vi "DAQ.vi"() -> ()   [LabVIEW 2014]
uses:
  <vilib>/LabVIEW Open Source Project/MQTT Control Packets/Control Packets/CONNECT/ConnectFlags -- cluster.ctl
  <vilib>/LabVIEW Open Source Project/MQTT Client/Client class/Client.lvclass/Client.ctl
  <vilib>/LabVIEW Open Source Project/MQTT Connection/MQTT_Base/Base Class/MQTT_Base.lvclass/MQTT_Base.ctl
  <vilib>/Utility/error.llb/Error Cluster From Error Code.vi
  <vilib>/LabVIEW Open Source Project/MQTT Control Packets/Control Packets/PUBLISH/PUBLISH.lvclass
  <vilib>/LabVIEW Open Source Project/MQTT Client/Client class/Client.lvclass
  <vilib>/ErrorRing/Error Ring.xnode
  <vilib>/LabVIEW Open Source Project/MQTT Connection/MQTT_Base/Base Class/MQTT_Base.lvclass
  <vilib>/LabVIEW Open Source Project/MQTT TCP Connection/MQTT_TCP/Connection/TCPConnection.lvclass
  <vilib>/LabVIEW Open Source Project/MQTT Control Packets/Control Packets/CONNECT/CONNECT.lvclass
panel:
  out "Array":string[](array[string])
  out "Data from subscribe":string
  out "Array 3":bool[](array[boolean])
  out "Time":u32
  in  "MQTT":enum32{"MQTT configs", "Equipment"}(tab)
  in  "Connect Flags":T1[](array[typedef])=[{"Reserved"=FALSE, "Clean Session"=FALSE, "Will Flag"=FALSE, "Will QoS 1"=FALSE, "Will QoS 2"=FALSE, "Will Retain"=FALSE, "Password Flag"=FALSE, "User Name Flag"=TRUE}, {"Reserved"=FALSE, "Clean Session"=FALSE, "Will Flag"=FALSE, "Will QoS 1"=FALSE, "Will QoS 2"=FALSE, "Will Retain"=FALSE, "Password Flag"=FALSE, "User Name Flag"=TRUE}, {"Reserved"=FALSE, "Clean Session"=FALSE, "Will Flag"=FALSE, "Will QoS 1"=FALSE, "Will QoS 2"=FALSE, "Will Retain"=FALSE, "Password Flag"=FALSE, "User Name Flag"=TRUE}, {"Reserved"=FALSE, "Clean Session"=FALSE, "Will Flag"=FALSE, "Will QoS 1"=FALSE, "Will QoS 2"=FALSE, "Will Retain"=FALSE, "Password Flag"=FALSE, "User Name Flag"=TRUE}, {"Reserved"=FALSE, "Clean Session"=FALSE, "Will Flag"=FALSE, "Will QoS 1"=FALSE, "Will QoS 2"=FALSE, "Will Retain"=FALSE, "Password Flag"=FALSE, "User Name Flag"=TRUE}, {"Reserved"=FALSE, "Clean Session"=FALSE, "Will Flag"=FALSE, "Will QoS 1"=FALSE, "Will QoS 2"=FALSE, "Will Retain"=FALSE, "Password Flag"=FALSE, "User Name Flag"=TRUE}]
  in  "User Devices":T2(array[cluster])=[{"Will Topic"="v1/devices/me/telemetry", "Will Message"="", "Username"="Valve-01", "Password"=""}, {"Will Topic"="v1/devices/me/telemetry", "Will Message"="", "Username"="Valve-02", "Password"=""}, {"Will Topic"="v1/devices/me/telemetry", "Will Message"="", "Username"="PP-01", "Password"=""}, {"Will Topic"="v1/devices/me/telemetry", "Will Message"="", "Username"="Level-01", "Password"=""}, {"Will Topic"="v1/devices/me/telemetry", "Will Message"="", "Username"="QT-01", "Password"=""}, {"Will Topic"="v1/devices/me/telemetry", "Will Message"="", "Username"="QT-02", "Password"=""}]
  in  "address (localhost)":string="things.ktk.gubkin.ru"
  in  "remote port (80)":u16=1883
  in  "PVs":string[](array[string])=["AI_rOpen_vlv1", "AI_rOpen_vlv2", "RA_rCntrl_engine_S", "AI_rlvl", "PV_AIFLOW1", "PV_AIFLOW2"]
  in  "OPs":string[](array[string])=["RA_rCntrl_vlv1_S", "RA_rCntrl_vlv2_S", "RA_rCntrl_engine_S"]
  out "error out":errorcluster
  in  "Frequency":dbl=10.0
  out "Display":string
  in  "Stop":bool
  in  "Exit":bool
  in  "Start":bool
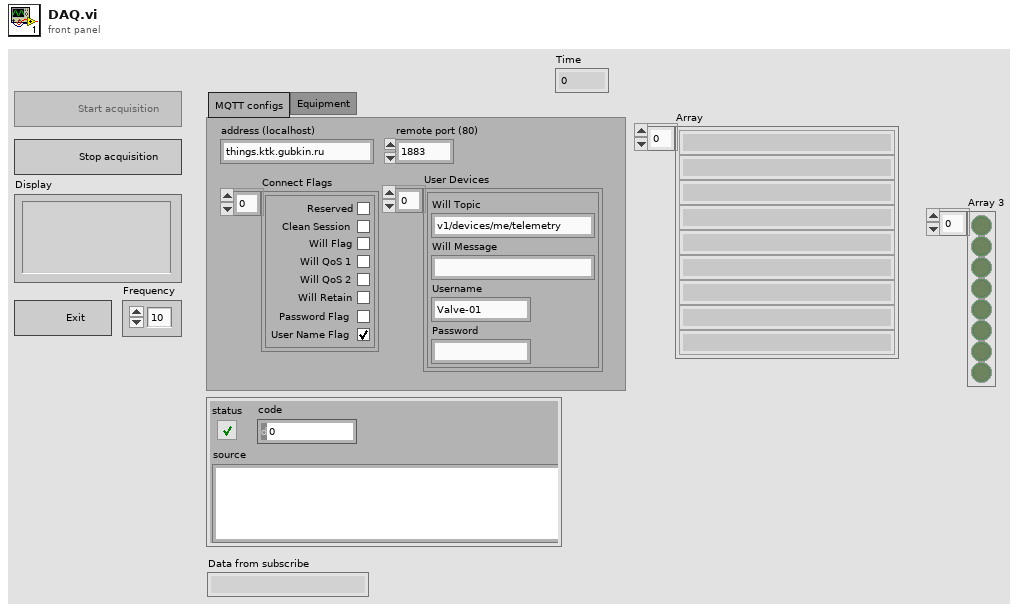
[diagram p1: front panel]
types:
  T1 = typedef "MQTT_Control_Packets.lvlib/CONNECT.lvclass/ConnectFlags -- cluster.ctl" = cluster{"Reserved":bool, "Clean Session":bool, "Will Flag":bool, "Will QoS 1":bool, "Will QoS 2":bool, "Will Retain":bool, "Password Flag":bool, "User Name Flag":bool}
  T2 = cluster{"Will Topic":string, "Will Message":string, "Username":string, "Password":string}[]
  T3 = cluster{"Start":refnum<vi>, "Stop":refnum<vi>, "Display":refnum<vi>, "Exit":refnum<vi>}
  T4 = cluster{"UI":refnum<queue>, "Acquisition":refnum<queue>}
  T5 = enum8{"Enabled", "Disabled", "Disabled and Grayed Out"}
  T6 = enum16{"Read", "Write", "ReadWrite", "BufferedRead", "BufferedReadWrite"}
  T7 = typedef "MQTT Client.lvlib/Client.lvclass/Public Events -- cluster.ctl" = cluster{"Connection Status":refnum<user-event>, "Connected":refnum<user-event>, "Application Message":refnum<user-event>}
  T8 = typedef "MQTT Base.lvlib/MQTT_Base.lvclass/Public Events -- cluster.ctl" = cluster{"Stop Event":refnum<user-event>, "Error Event":refnum<user-event>, "Inbound Message":refnum<user-event>}
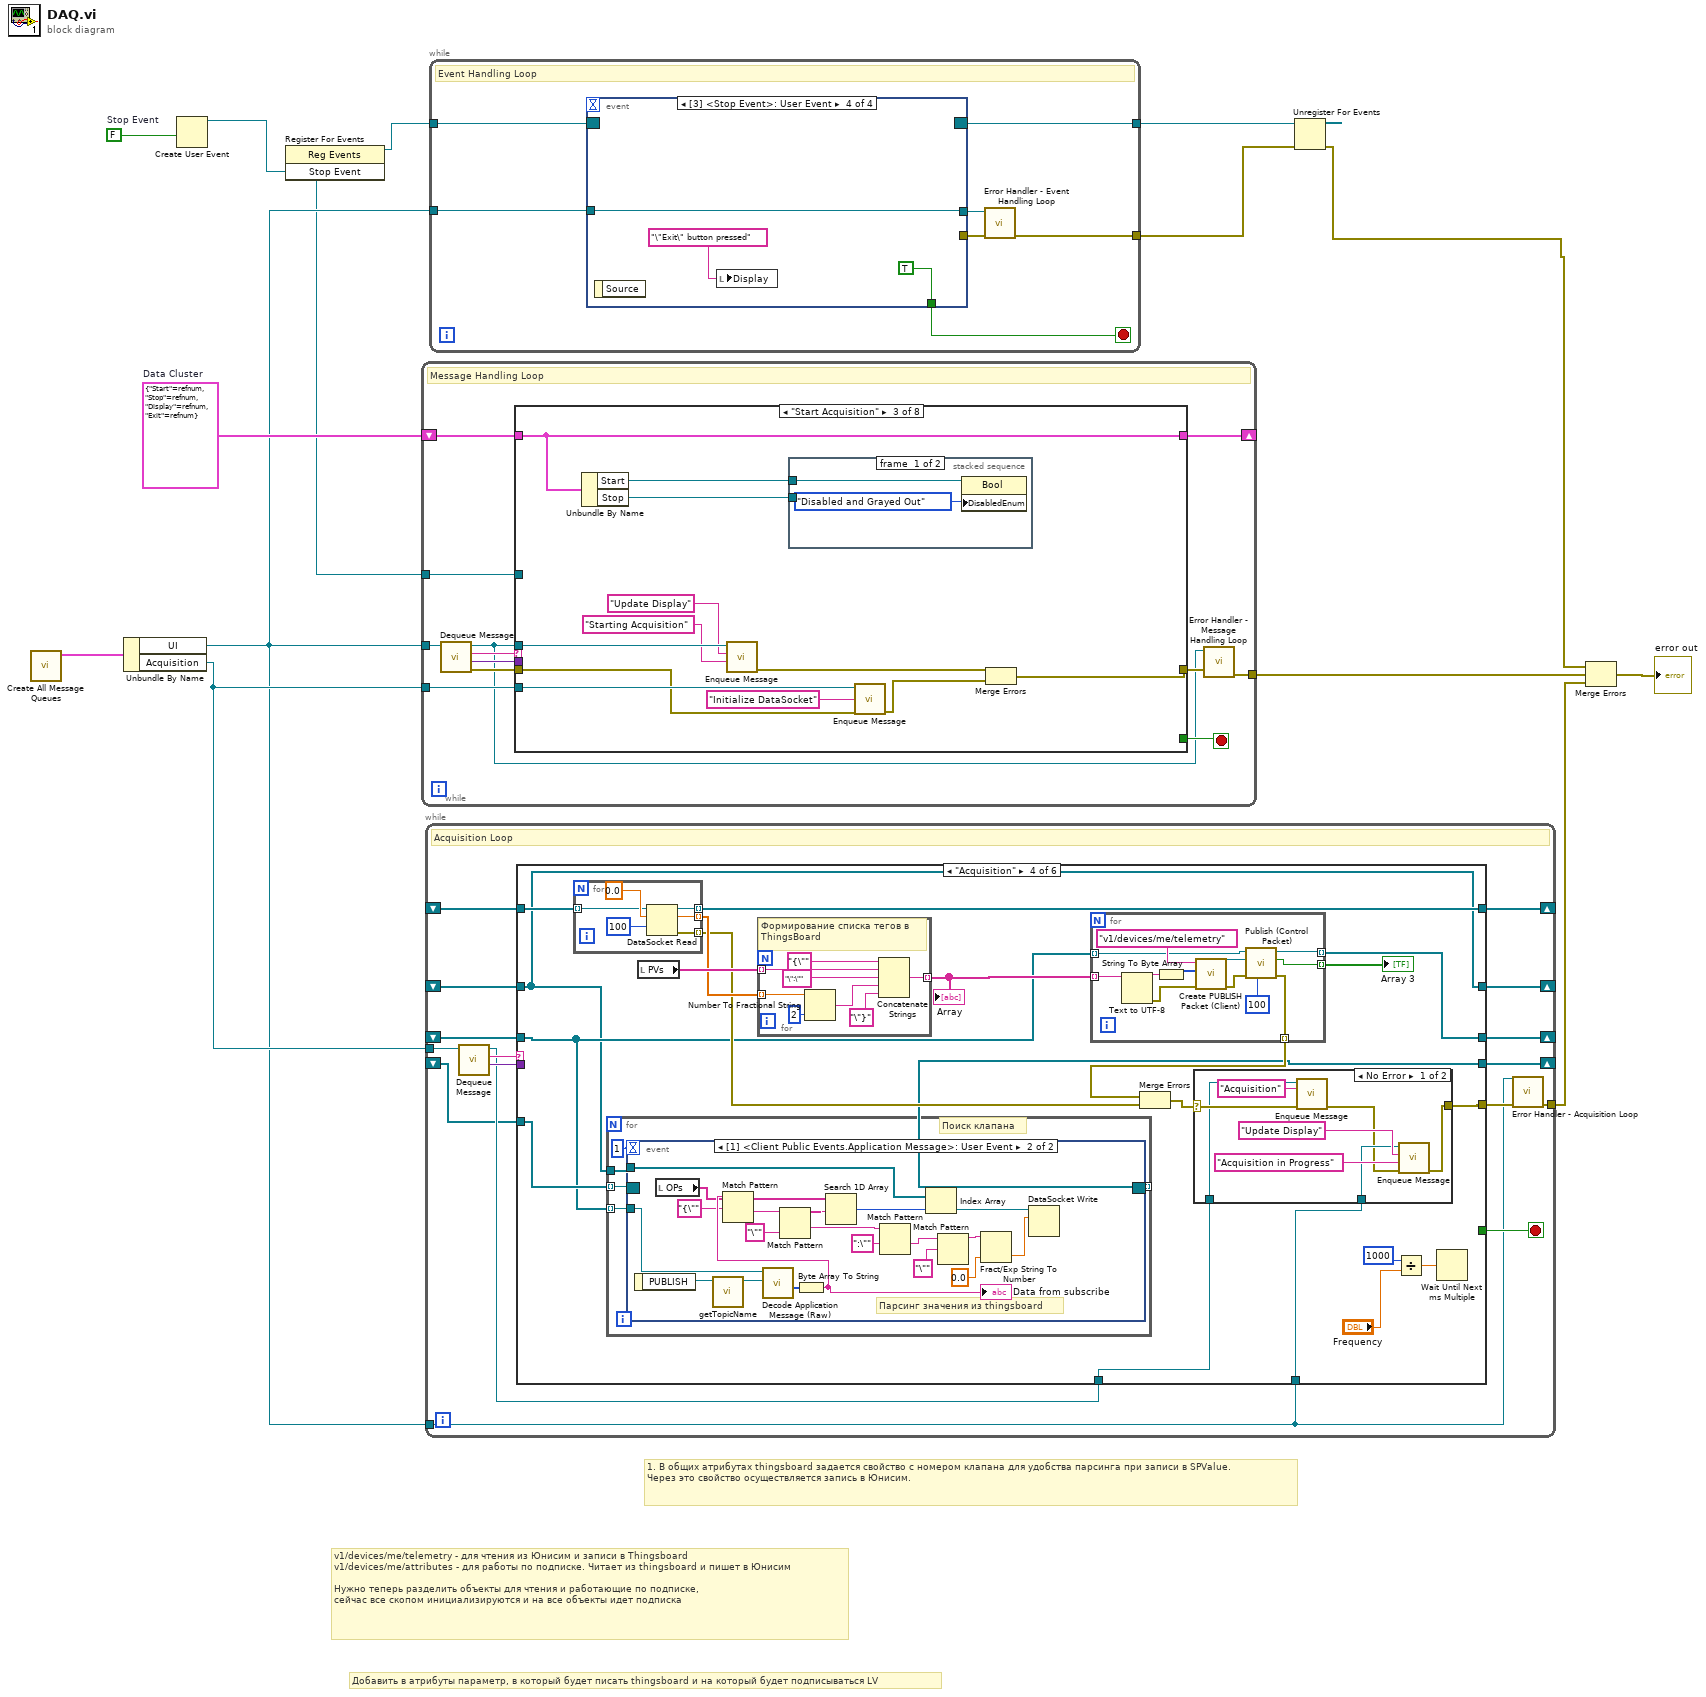
[diagram p0: block diagram]
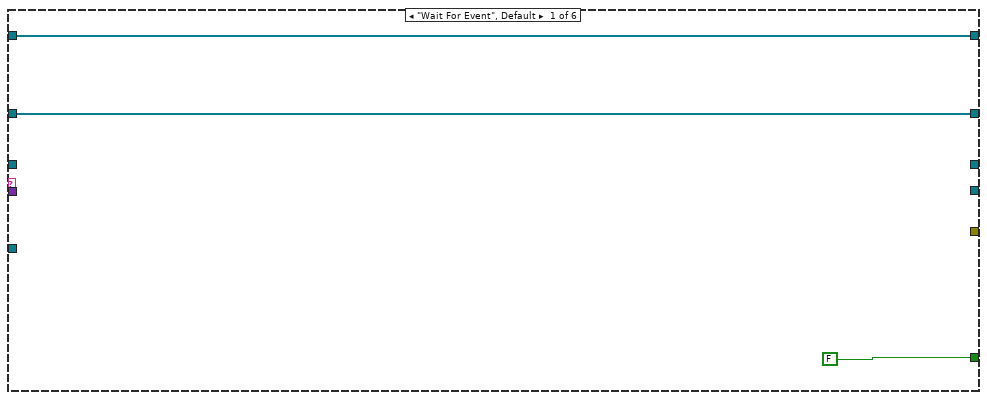
[diagram p2: hidden frame]
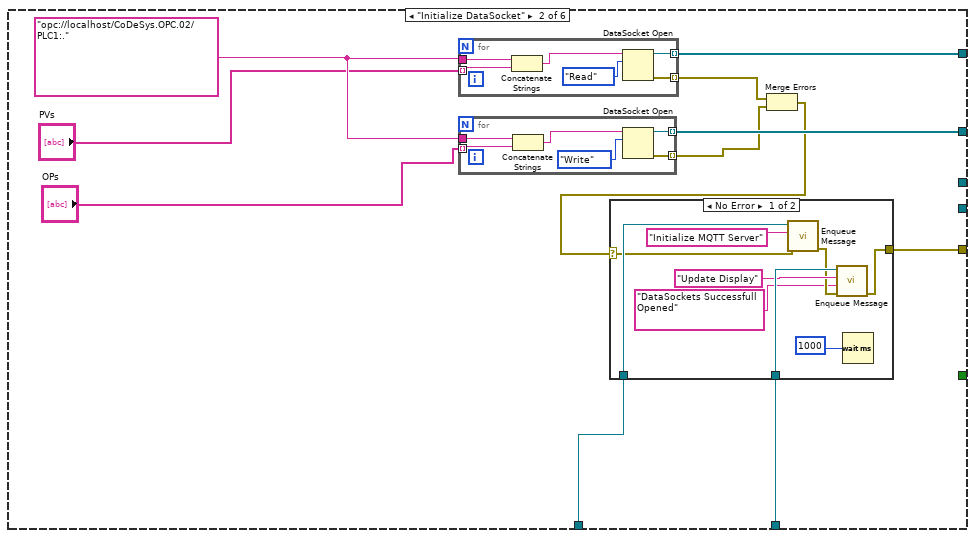
[diagram p3: hidden frame]
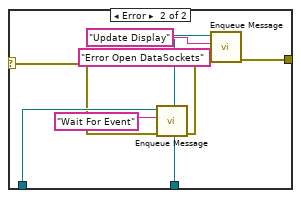
[diagram p4: hidden frame]
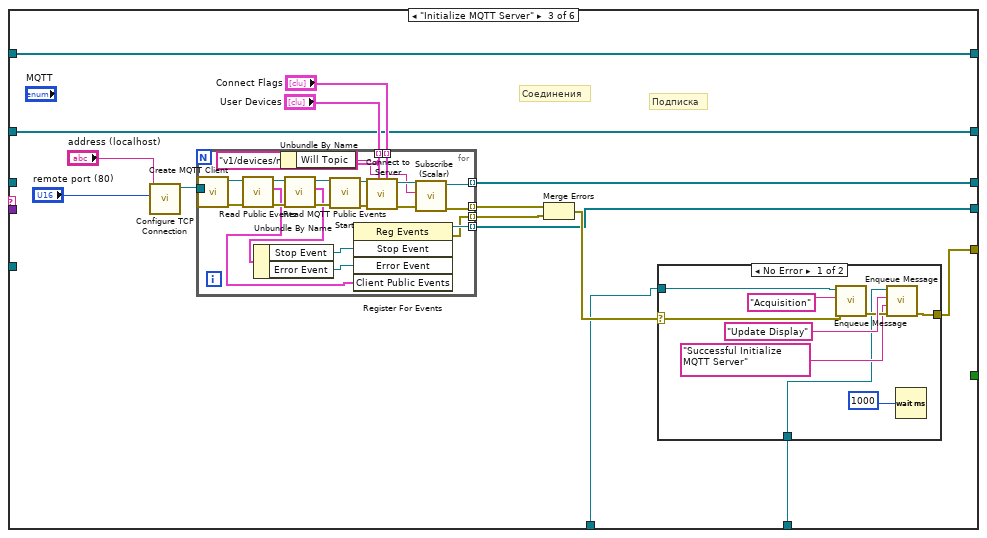
[diagram p5: hidden frame]
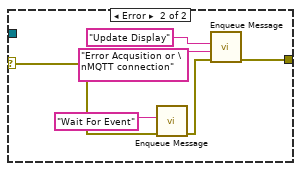
[diagram p6: hidden frame]
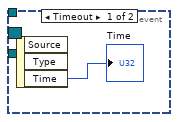
[diagram p7: hidden frame]
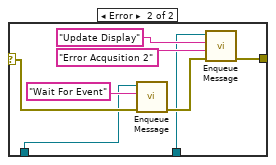
[diagram p8: hidden frame]
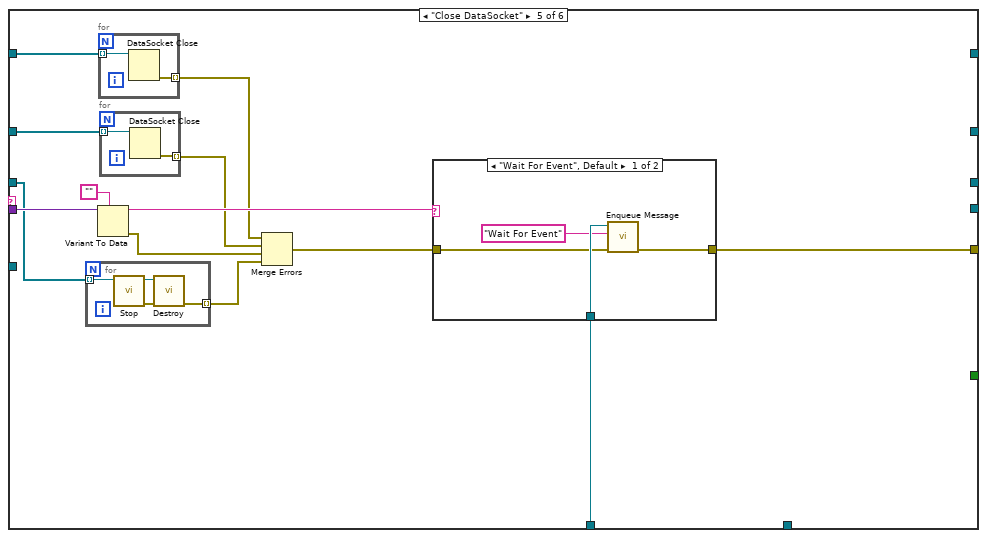
[diagram p9: hidden frame]
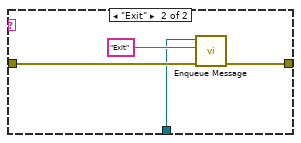
[diagram p10: hidden frame]
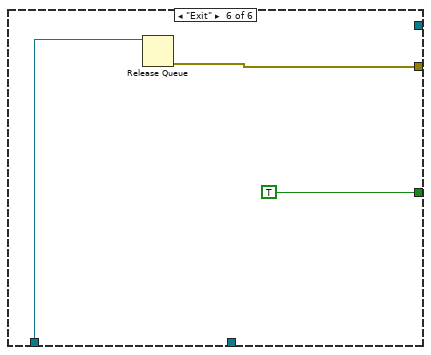
[diagram p11: hidden frame]
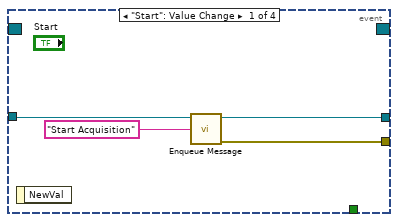
[diagram p12: hidden frame]
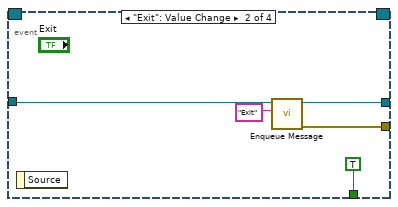
[diagram p13: hidden frame]
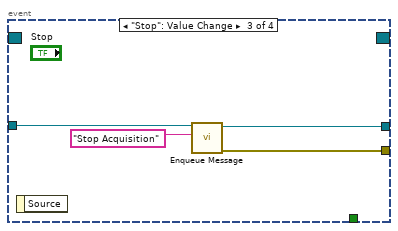
[diagram p14: hidden frame]
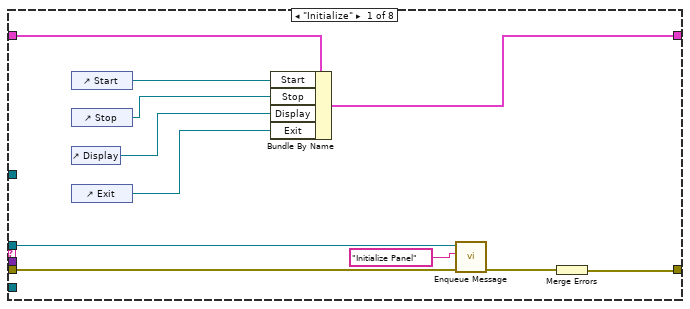
[diagram p15: hidden frame]
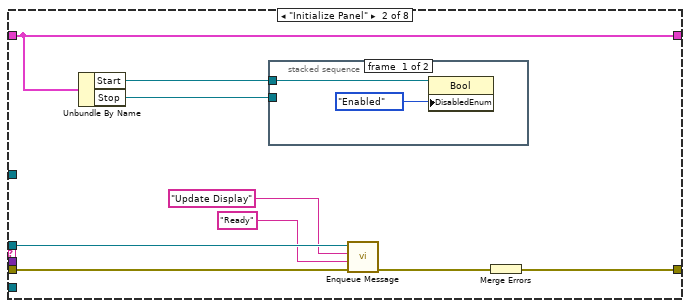
[diagram p16: hidden frame]
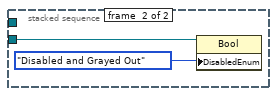
[diagram p17: hidden frame]
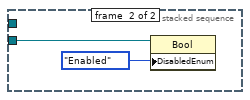
[diagram p18: hidden frame]
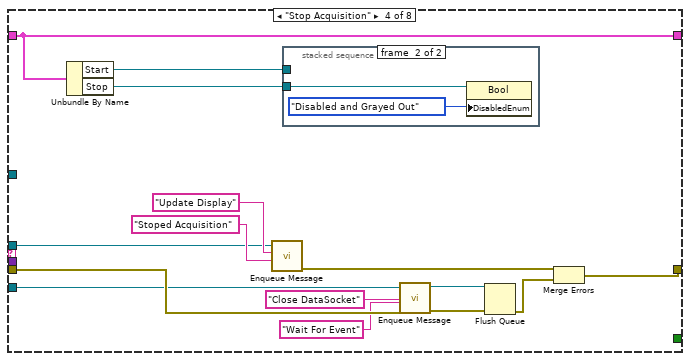
[diagram p19: hidden frame]
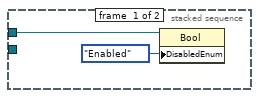
[diagram p20: hidden frame]
diagram:
  w7 = FALSE  # Stop Event
  w12 = T3 {"Start"=refnum, "Stop"=refnum, "Display"=refnum, "Exit"=refnum}  # Data Cluster
  # "1. В общих атрибутах thingsboard задается свойство с номером клапана для удобства парсинга при записи в SPValue.\nЧерез это свойство осуществляется запись в Юнисим."
  # "Добавить в атрибуты параметр, в который будет писать thingsboard и на который будет подписываться LV"
  # "v1/devices/me/telemetry - для чтения из Юнисим и записи в Thingsboard\nv1/devices/me/attributes - для работы по подписке. Читает из thingsboard и пишет в Юнисим\n\nНужно теперь разделить объекты для чтения и работающие по подписке,\nсейчас все скопом инициализируются и на все объекты идет подписка"
  n1 = call "Create All Message Queues.vi"() -> ("Message Queues out"=w13:T4)  [unwired: 10 in, 1 out]
  n2 = Unbundle By Name(w13) -> ("UI"=w10:refnum<queue>, "Acquisition"=w11:refnum<queue>)
  n3 = Create User Event(user event datatype=w7) -> (user event=w6:refnum<user-event>)  [unwired: 1 in, 1 out]
  n4 = register-events(w6) -> (reference out=w5:refnum<event-registration>)  [unwired: 2 in, 1 out]
  n5 = while {
    tunnel: w10 -> [w24]
    shift-right: [w22] -> _
    shift-left: w12 -> [w18]
    tunnel: w11 -> [w21]
    tunnel: [w16] -> w9
    tunnel: w6 -> [w14]
    stop <- w19 stop-if-true
    # "Message Handling Loop"
    n6 = call "Dequeue Message.vi"("Queue in"=w24) -> ("error out"=w23:errorcluster, "Message Data"=w20:variant, "Message"=w25:string, "Queue out"=w15:refnum<queue>)  [unwired: 7 in]
    n7 = case shown="\"Start Acquisition\"" w25 {
      selector: w25 -> [_ _ _ _ _ _ _ w121]
      tunnel: w18 -> [w36 w44 w61 w80 w88 w93 w115 w122]
      tunnel: w15 -> [w31 w43 w58 w73 _ w98 w112 _]
      tunnel: w23 -> [w30 w42 w51 w72 w89 w100 w111 _]
      tunnel: [w28 w44 w61 w80 w88 w93 w115 w122] -> w22
      tunnel: w21 -> [_ _ w55 w71 _ _ w110 _]
      tunnel: w20 -> [_ _ _ _ w90 w101 _ _]
      tunnel: [_ _ _ _ _ _ TRUE _] -> w19
      tunnel: [w26 w37 w50 w66 w85 w92 w104 w120] -> w17
      tunnel: w14 -> [_ _ _ _ _ _ w103 _]
      frame "Initialize" {
        n8 = control-ref of="Start"() -> (w35:refnum<vi>)
        n9 = control-ref of="Stop"() -> (w34:refnum<vi>)
        n10 = control-ref of="Display"() -> (w33:refnum<vi>)
        n11 = control-ref of="Exit"() -> (w32:refnum<vi>)
        n12 = Bundle By Name(cluster=w36, "Start"=w35, "Stop"=w34, "Display"=w33, "Exit"=w32) -> (w28:T3)
        n13 = call "Enqueue Message.vi"("error in (no error)"=w30, "Message"="Initialize Panel", "Queue in"=w31) -> ("error out"=w27:errorcluster)  [unwired: 7 in, 1 out]
        n14 = Merge Errors(w27) -> (w26:errorcluster)
      }
      frame "Initialize Panel" {
        n15 = Unbundle By Name(w44) -> ("Start"=w38:refnum<vi>, "Stop"=w45:refnum<vi>)
        n16 = stacked-sequence {
          tunnel: w38 -> [w47 _]
          tunnel: w45 -> [_ w48]
          frame #0 {
            n17 = property class="Bool"(reference=w47, "DisabledEnum"=T5."Enabled" ("Disabled")) -> ()  [unwired: 1 in, 2 out]
          }
          frame #1 {
            n18 = property class="Bool"(reference=w48, "DisabledEnum"=T5."Disabled and Grayed Out" ("Disabled")) -> ()  [unwired: 1 in, 2 out]
          }
        }
        n19 = call "Enqueue Message.vi"("error in (no error)"=w42, "Message Data"="Ready" ("Message"), "Message"="Update Display", "Queue in"=w43) -> ("error out"=w39:errorcluster)  [unwired: 6 in, 1 out]
        n20 = Merge Errors(w39) -> (w37:errorcluster)
      }
      frame "Start Acquisition" {
        n21 = Unbundle By Name(w61) -> ("Start"=w60:refnum<vi>, "Stop"=w59:refnum<vi>)
        n22 = call "Enqueue Message.vi"("Message Data"="Starting Acquisition" ("Message"), "Message"="Update Display", "Queue in"=w58) -> ("error out"=w53:errorcluster)  [unwired: 7 in, 1 out]
        n23 = stacked-sequence {
          tunnel: w60 -> [w62 _]
          tunnel: w59 -> [_ w64]
          frame #0 {
            n24 = property class="Bool"(reference=w62, "DisabledEnum"=T5."Disabled and Grayed Out" ("Disabled")) -> ()  [unwired: 1 in, 2 out]
          }
          frame #1 {
            n25 = property class="Bool"(reference=w64, "DisabledEnum"=T5."Enabled" ("Disabled")) -> ()  [unwired: 1 in, 2 out]
          }
        }
        n26 = call "Enqueue Message.vi"("error in (no error)"=w51, "Message"="Initialize DataSocket", "Queue in"=w55) -> ("error out"=w52:errorcluster)  [unwired: 7 in, 1 out]
        n27 = Merge Errors(w53, w52) -> (w50:errorcluster)
      }
      frame "Stop Acquisition" {
        n28 = Unbundle By Name(w80) -> ("Start"=w79:refnum<vi>, "Stop"=w78:refnum<vi>)
        n29 = call "Enqueue Message.vi"("Message Data"="Stoped Acquisition" ("Message"), "Message"="Update Display", "Queue in"=w73) -> ("error out"=w77:errorcluster)  [unwired: 7 in, 1 out]
        n30 = stacked-sequence {
          tunnel: w79 -> [w81 _]
          tunnel: w78 -> [_ w83]
          frame #0 {
            n31 = property class="Bool"(reference=w81, "DisabledEnum"=T5."Enabled" ("Disabled")) -> ()  [unwired: 1 in, 2 out]
          }
          frame #1 {
            n32 = property class="Bool"(reference=w83, "DisabledEnum"=T5."Disabled and Grayed Out" ("Disabled")) -> ()  [unwired: 1 in, 2 out]
          }
        }
        n33 = call "Enqueue Message.vi"("error in (no error)"=w72, "Message Data"="Wait For Event" ("Message"), "Message"="Close DataSocket", "Queue in"=w71) -> ("error out"=w68:errorcluster, "Queue out"=w69:refnum<queue>)  [unwired: 6 in]
        n34 = Flush Queue(queue=w69, error in (no error)=w68) -> (error out=w67:errorcluster)  [unwired: 2 out]
        n35 = Merge Errors(w77, w67) -> (w66:errorcluster)
      }
      frame "Update Display" {
        n36 = Variant To Data(error in=w89, type="", Variant=w90) -> (data=→"Display":string, error out=w86:errorcluster)
        n37 = Merge Errors(w86) -> (w85:errorcluster)
      }
      frame "Error" {
        n38 = Variant To Data(error in=w100, Variant=w101) -> (data=w99:errorcluster, error out=w94:errorcluster)  [unwired: 1 in]
        n39 = call <vilib>:"Simple Error Handler.vi"("error in (no error)"=w99) -> ()  [unwired: 4 in, 5 out]
        n40 = call "Enqueue Message.vi"("Priority Message"=TRUE, "Message"="Exit", "Queue in"=w98) -> ("error out"=w95:errorcluster)  [unwired: 7 in, 1 out]
        n41 = Merge Errors(w95, w94) -> (w92:errorcluster)
      }
      frame "Exit" {
        n42 = Unbundle By Name(w115) -> ("Start"=w114:refnum<vi>, "Stop"=w113:refnum<vi>)
        n43 = Release Queue(queue=w112, error in (no error)=w111) -> (error out=w106:errorcluster)  [unwired: 1 in, 2 out]
        n44 = Generate User Event(user event=w103, event data cluster=TRUE ("event data")) -> ()  [unwired: 2 in, 2 out]
        n45 = call "Enqueue Message.vi"("Message Data"="Exit" ("Message"), "Message"="Close DataSocket", "Queue in"=w110) -> ("error out"=w107:errorcluster)  [unwired: 7 in, 1 out]
        n46 = stacked-sequence {
          tunnel: w114 -> [w116 _]
          tunnel: w113 -> [_ w118]
          frame #0 {
            n47 = property class="Bool"(reference=w116, "DisabledEnum"=T5."Enabled" ("Disabled")) -> ()  [unwired: 1 in, 2 out]
          }
          frame #1 {
            n48 = property class="Bool"(reference=w118, "DisabledEnum"=T5."Disabled and Grayed Out" ("Disabled")) -> ()  [unwired: 1 in, 2 out]
          }
        }
        n49 = Merge Errors(w106, w107) -> (w104:errorcluster)
      }
      frame Default {
        n50 = xnode "Error Ring"("parameter 0"=w121) -> ("error out"=w120:errorcluster)
      }
    }
    n51 = call "Error Handler - Message Handling Loop.vi"("error in (no error)"=w17, "Message Queue"=w15) -> ("dup error in"=w16:errorcluster)  [unwired: 8 in, 1 out]
  }
  n52 = while {
    tunnel: w11 -> [w144]
    shift-right: [w143] -> _
    shift-left: _ -> [w141]
    shift-right: [w142] -> _
    shift-left: _ -> [w140]
    tunnel: w10 -> [w134]
    tunnel: [w136] -> w1
    shift-right: [w133] -> _
    shift-left: _ -> [w132]
    shift-right: [w131] -> _
    shift-left: _ -> [w130]
    stop <- w135 stop-if-true
    # "Acquisition Loop"
    n53 = call "Dequeue Message.vi"("Queue in"=w144) -> ("Message Data"=w139:variant, "Message"=w145:string, "Queue out"=w138:refnum<queue>)  [unwired: 7 in, 1 out]
    n54 = case shown="\"Acquisition\"" w145 {
      tunnel: [w148 w158 w198 w258 _ _] -> w143
      tunnel: [w147 w157 w197 w241 _ _] -> w142
      tunnel: w141 -> [w148 _ w198 w259 w338 _]
      tunnel: w140 -> [w147 _ w197 w241 w337 _]
      tunnel: w138 -> [_ w154 w192 w252 w336 w360]
      tunnel: w139 -> [_ _ _ _ w340 _]
      tunnel: w134 -> [_ w153 w191 w253 _ _]
      tunnel: [_ w152 w193 w254 w331 w359] -> w137
      tunnel: [FALSE _ _ _ _ TRUE] -> w135
      tunnel: [_ _ w196 w243 _ _] -> w133
      tunnel: w132 -> [_ _ _ w245 w330 _]
      tunnel: [_ _ w190 w244 _ _] -> w131
      tunnel: w130 -> [_ _ _ w246 _ _]
      frame "Wait For Event", Default {
      }
      frame "Initialize DataSocket" {
        w159 = "opc://localhost/CoDeSys.OPC.02/PLC1:."
        n55 = for {
          tunnel: w159 -> [w188]
          tunnel: "PVs" -> [w185] mode=indexing
          tunnel: [w184] -> w158 mode=indexing
          tunnel: [w183] -> w156 mode=indexing
          n56 = Concatenate Strings(w188, w185) -> (w186:string)
          n57 = DataSocket Open(10:T6."Read" ("mode"), 11:w186) -> (0:w183:errorcluster, 3:w184:refnum<k13>)  [unwired: 2 in]
        }
        n58 = for {
          tunnel: w159 -> [w165]
          tunnel: "OPs" -> [w163] mode=indexing
          tunnel: [w162] -> w157 mode=indexing
          tunnel: [w161] -> w155 mode=indexing
          n59 = Concatenate Strings(w165, w163) -> (w160:string)
          n60 = DataSocket Open(10:T6."Write" ("mode"), 11:w160) -> (0:w161:errorcluster, 3:w162:refnum<k13>)  [unwired: 2 in]
        }
        n61 = Merge Errors(w156, w155) -> (w151:errorcluster)
        n62 = case shown="No Error" w151 {
          selector: w151 -> [w172 w178]
          tunnel: w154 -> [w173 w182]
          tunnel: w153 -> [w171 w179]
          tunnel: [w168 w176] -> w152
          frame No Error {
            n63 = call "Enqueue Message.vi"("error in (no error)"=w172, "Message"="Initialize MQTT Server", "Queue in"=w173) -> ("error out"=w169:errorcluster)  [unwired: 7 in, 1 out]
            n64 = call "Enqueue Message.vi"("error in (no error)"=w169, "Message Data"="DataSockets Successfull Opened" ("Message"), "Message"="Update Display", "Queue in"=w171) -> ("error out"=w168:errorcluster)  [unwired: 6 in, 1 out]
            n65 = Wait (ms)(milliseconds to wait=u32 1000) -> ()  [unwired: 1 out]
          }
          frame Error {
            n66 = call "Enqueue Message.vi"("error in (no error)"=w178, "Message"="Wait For Event", "Queue in"=w182) -> ("error out"=w175:errorcluster)  [unwired: 7 in, 1 out]
            n67 = call "Enqueue Message.vi"("error in (no error)"=w175, "Message Data"="Error Open DataSockets", "Message"="Update Display", "Queue in"=w179) -> ("error out"=w176:errorcluster)  [unwired: 6 in, 1 out]
          }
        }
      }
      frame "Initialize MQTT Server" {
        # "Соединения"
        # "Подписка"
        n68 = call <vilib>:"Configure TCP Connection.vi"("remote port (80)"="remote port (80)", "address (localhost)"="address (localhost)") -> ("TCPConnection"=w201:refnum<class "TCPConnection.lvclass">)  [unwired: 8 in, 1 out]
        n69 = for {
          tunnel: w201 -> [w239]
          tunnel: "Connect Flags" -> [w221] mode=indexing
          tunnel: "User Devices" -> [w220] mode=indexing
          tunnel: [w223] -> w196 mode=indexing
          tunnel: [w222] -> w195 mode=indexing
          tunnel: [w227] -> w190 mode=indexing
          tunnel: [w226] -> w189 mode=indexing
          n70 = call <vilib>:"Create MQTT Client.vi"("Connection Configuration"=w239) -> ("error out"=w234:errorcluster, "Client out"=w237:refnum<class "Client.lvclass">)  [unwired: 9 in]
          n71 = call <vilib>:"Read Public Events.vi"("error in (no error)"=w234, "Client in"=w237) -> ("error out"=w233:errorcluster, "Client Public Events"=w228:T7, "Client out"=w236:refnum<class "Client.lvclass">)  [unwired: 7 in]
          n72 = Unbundle By Name(w220) -> ()  [unwired: 1 out]
          n73 = call <vilib>:"Read MQTT Public Events.vi"("error in (no error)"=w233, "MQTT_Base in"=w236) -> ("error out"=w232:errorcluster, "MQTT Public Events"=w231:T8, "MQTT_Base out"=w235:refnum<class "Client.lvclass">)  [unwired: 7 in]
          n74 = Unbundle By Name(w231) -> ("Stop Event"=w230:refnum<user-event>, "Error Event"=w229:refnum<user-event>)
          n75 = call <vilib>:"Start.vi"("error in (no error)"=w232, "MQTT_Base in"=w235) -> ("error out"=w240:errorcluster, "MQTT_Base out"=w238:refnum<class "Client.lvclass">)  [unwired: 7 in, 1 out]
          n76 = register-events(w230, w229, w228) -> (reference out=w227:refnum<event-registration>, error out=w226:errorcluster)  [unwired: 2 in]
          n77 = call <vilib>:"Connect to Server.vi"("Connect Flags"=w221, "Payload"=w220, "error in (no error)"=w240, "Client in"=w238) -> ("error out"=w224:errorcluster, "Client out"=w225:refnum<class "Client.lvclass">)  [unwired: 4 in, 2 out]
          n78 = call <vilib>:"Subscribe (Scalar).vi"("error in (no error)"=w224, "Topic Filter"="v1/devices/me/attributes" ("Topic Name (empty: Payload name)"), "Client in"=w225) -> ("error out"=w222:errorcluster, "Client out"=w223:refnum<class "Client.lvclass">)  [unwired: 6 in, 1 out]
        }
        n79 = Merge Errors(w195, w189) -> (w194:errorcluster)
        n80 = case shown="No Error" w194 {
          selector: w194 -> [w211 w216]
          tunnel: [w208 w214] -> w193
          tunnel: w192 -> [w205 _]
          tunnel: w191 -> [w204 _]
          frame No Error {
            n81 = call "Enqueue Message.vi"("error in (no error)"=w211, "Message"="Acquisition", "Queue in"=w205) -> ("error out"=w209:errorcluster)  [unwired: 7 in, 1 out]
            n82 = call "Enqueue Message.vi"("error in (no error)"=w209, "Message Data"="Successful Initialize MQTT Server" ("Message"), "Message"="Update Display", "Queue in"=w204) -> ("error out"=w208:errorcluster)  [unwired: 6 in, 1 out]
            n83 = Wait (ms)(milliseconds to wait=u32 1000) -> ()  [unwired: 1 out]
          }
          frame Error {
            n84 = call "Enqueue Message.vi"("error in (no error)"=w216, "Message"="Wait For Event") -> ("error out"=w213:errorcluster)  [unwired: 8 in, 1 out]
            n85 = call "Enqueue Message.vi"("error in (no error)"=w213, "Message Data"="Error Acqusition or \nMQTT connection", "Message"="Update Display") -> ("error out"=w214:errorcluster)  [unwired: 7 in, 1 out]
          }
        }
      }
      frame "Acquisition" {
        n86 = for {
          tunnel: w259 -> [w327] mode=indexing
          tunnel: [w326] -> w258 mode=indexing
          tunnel: [w325] -> w250 mode=indexing
          tunnel: [w323] -> w248 mode=indexing
          n87 = DataSocket Read(9:100 ("ms timeout (10000)"), 10:0.0, 11:w327) -> (0:w323:errorcluster, 2:w325:dbl, 3:w326:refnum<k13>)  [unwired: 2 in, 4 out]
        }
        n88 = for {
          tunnel: w246 -> [w265] mode=indexing
          tunnel: w245 -> [w264] mode=indexing
          tunnel: [w262] -> w244 mode=indexing
          tunnel: w241 -> [w261]
          # "Поиск клапана"
          n89 = event shown="[1] <Client Public Events.Application Message>: User Event" {
            selector: w265 -> [_ _]
            dyn-events: [_ _] -> w262
            timeout: 1 -> [_ _]
            tunnel: w264 -> [_ w283]
            tunnel: w261 -> [_ w271]
            event Timeout {
              n90 = event-data() -> ("Time"=→"Time":u32)  [unwired: 1 in, 2 out]
            }
            event User Event {
              # "Парсинг значения из thingsboard"
              n91 = event-data() -> ("PUBLISH"=w284:refnum<class "PUBLISH.lvclass">)  [unwired: 1 in]
              n92 = local read "OPs"() -> (w274:string[])
              n93 = call <vilib>:"getTopicName.vi"("PUBLISH in"=w284) -> ("PUBLISH out"=w285:refnum<class "PUBLISH.lvclass">)  [unwired: 8 in, 2 out]
              n94 = call <vilib>:"Decode Application Message (Raw).vi"("PUBLISH"=w285, "Client in"=w283) -> ("Payload"=w286:u8[])  [unwired: 6 in, 3 out]
              n95 = Byte Array To String(unsigned byte array=w286) -> (string=w282:string)
              "Data from subscribe" <- w282
              n96 = Match Pattern(string=w282, regular expression="{\"") -> (after substring=w280:string)  [unwired: 1 in, 3 out]
              n97 = Match Pattern(string=w280, regular expression="\"") -> (before substring=w273:string, after substring=w278:string)  [unwired: 1 in, 2 out]
              n98 = Search 1D Array(1D array=w274, element=w273) -> (index of element=w270:i32)  [unwired: 1 in]
              n99 = Match Pattern(string=w278, regular expression=":\"") -> (after substring=w276:string)  [unwired: 1 in, 3 out]
              n100 = Index Array(array=w271, index=w270) -> (element=w272:refnum<k13>)
              n101 = Match Pattern(string=w276, regular expression="\"") -> (before substring=w268:string)  [unwired: 1 in, 3 out]
              n102 = Fract/Exp String To Number(string=w268, default (0 dbl)=0.0 ("default (0 I32)")) -> (number=w267:dbl)  [unwired: 2 in, 1 out]
              n103 = DataSocket Write(10:w267, 11:w272) -> ()  [unwired: 2 in, 3 out]
            }
          }
        }
        n104 = local read "PVs"() -> (w251:string[])
        n105 = for {
          tunnel: w251 -> [w305] mode=indexing
          tunnel: w250 -> [w303] mode=indexing
          tunnel: [w299] -> w249 mode=indexing
          # "Формирование списка тегов в ThingsBoard"
          n106 = Number To Fractional String(number=w303, precision (6)=i16 2) -> (F-format string=w302:string)  [unwired: 2 in]
          n107 = Concatenate Strings("{\"" ("string"), w305, "\":\"" ("string"), w302, "\"}" ("string")) -> (w299:string)
        }
        "Array" <- w249
        n108 = for {
          tunnel: w249 -> [w293] mode=indexing
          tunnel: w245 -> [w290] mode=indexing
          tunnel: [w289] -> w247 mode=indexing
          tunnel: [w288] -> w243 mode=indexing
          tunnel: [w287] -> w242 mode=indexing
          n109 = Text to UTF-8(11:w293) -> (0:w294:errorcluster, 3:w296:string)  [unwired: 2 in]
          n110 = String To Byte Array(string=w296) -> (unsigned byte array=w295:u8[])
          n111 = call <vilib>:"Create PUBLISH Packet (Client).vi"("error in (no error)"=w294, "Payload"=w295, "Topic Name"="v1/devices/me/telemetry" ("Topic Name (empty: Payload name)")) -> ("error out"=w292:errorcluster, "PUBLISH"=w297:refnum<class "PUBLISH.lvclass">)  [unwired: 5 in, 2 out]
          n112 = call <vilib>:"Publish (Control Packet).vi"("timeout (1000ms)"=100 ("timeout (0ms : no ack)"), "error in (no error)"=w292, "PUBLISH"=w297, "Client in"=w290) -> ("error out"=w289:errorcluster, "Published"=w287:bool, "Client out"=w288:refnum<class "Client.lvclass">)  [unwired: 5 in]
        }
        "Array 3" <- w242
        n113 = Merge Errors(w247, w248) -> (w255:errorcluster)
        n114 = case shown="No Error" w255 {
          selector: w255 -> [w313 w316]
          tunnel: w252 -> [w312 w315]
          tunnel: [w307 w317] -> w254
          tunnel: w253 -> [w309 w318]
          frame No Error {
            n115 = call "Enqueue Message.vi"("error in (no error)"=w313, "Message"="Acquisition", "Queue in"=w312) -> ("error out"=w308:errorcluster)  [unwired: 7 in, 1 out]
            n116 = call "Enqueue Message.vi"("error in (no error)"=w308, "Message Data"="Acquisition in Progress" ("Message"), "Message"="Update Display", "Queue in"=w309) -> ("error out"=w307:errorcluster)  [unwired: 6 in, 1 out]
          }
          frame Error {
            n117 = call "Enqueue Message.vi"("error in (no error)"=w316, "Message"="Wait For Event", "Queue in"=w315) -> ("error out"=w319:errorcluster)  [unwired: 7 in, 1 out]
            n118 = call "Enqueue Message.vi"("error in (no error)"=w319, "Message Data"="Error Acqusition 2", "Message"="Update Display", "Queue in"=w318) -> ("error out"=w317:errorcluster)  [unwired: 6 in, 1 out]
          }
        }
        n119 = Divide(x=u32 1000 ("millisecond multiple"), y="Frequency") -> (x/y=w257:dbl)
        n120 = Wait Until Next ms Multiple(millisecond multiple=w257) -> ()  [unwired: 1 out]
      }
      frame "Close DataSocket" {
        n121 = for {
          tunnel: w330 -> [w342] mode=indexing
          tunnel: [w343] -> w329 mode=indexing
          n122 = call <vilib>:"Stop.vi"("MQTT_Base in"=w342) -> ("error out"=w344:errorcluster, "MQTT_Base out"=w345:refnum<class "Client.lvclass">)  [unwired: 8 in, 1 out]
          n123 = call <vilib>:"Destroy.vi"("error in (no error)"=w344, "MQTT_Base in"=w345) -> ("error out"=w343:errorcluster)  [unwired: 8 in, 1 out]
        }
        n124 = Variant To Data(type="", Variant=w340) -> (data=w339:string, error out=w333:errorcluster)  [unwired: 1 in]
        n125 = for {
          tunnel: w338 -> [w349] mode=indexing
          tunnel: [w348] -> w335 mode=indexing
          n126 = DataSocket Close(11:w349) -> (0:w348:errorcluster)  [unwired: 2 in, 1 out]
        }
        n127 = for {
          tunnel: w337 -> [w347] mode=indexing
          tunnel: [w346] -> w334 mode=indexing
          n128 = DataSocket Close(11:w347) -> (0:w346:errorcluster)  [unwired: 2 in, 1 out]
        }
        n129 = Merge Errors(w335, w334, w333, w329) -> (w332:errorcluster)
        n130 = case shown="\"Wait For Event\", Default" w339 {
          tunnel: w336 -> [w353 w354]
          tunnel: w332 -> [w351 w356]
          tunnel: [w350 w355] -> w331
          frame "Wait For Event", Default {
            n131 = call "Enqueue Message.vi"("error in (no error)"=w351, "Message"="Wait For Event", "Queue in"=w353) -> ("error out"=w350:errorcluster)  [unwired: 7 in, 1 out]
          }
          frame "Exit" {
            n132 = call "Enqueue Message.vi"("error in (no error)"=w356, "Message"="Exit", "Queue in"=w354) -> ("error out"=w355:errorcluster)  [unwired: 7 in, 1 out]
          }
        }
      }
      frame "Exit" {
        n133 = Release Queue(queue=w360) -> (error out=w359:errorcluster)  [unwired: 2 in, 2 out]
      }
    }
    n134 = call "Error Handler - Acquisition Loop.vi"("error in (no error)"=w137, "Message Queue"=w134) -> ("dup error in"=w136:errorcluster)  [unwired: 8 in, 1 out]
  }
  n135 = while {
    tunnel: w10 -> [w367]
    tunnel: [w363] -> w3
    tunnel: w5 -> [w362]
    tunnel: [w361] -> w4
    stop <- w366 stop-if-true
    # "Event Handling Loop"
    n136 = event shown="[3] <Stop Event>: User Event" {
      selector: w362 -> [_ _ _ _]
      dyn-events: [_ _ _ _] -> w361
      timeout: _ -> [_ _ _ _]
      tunnel: w367 -> [w371 w375 w379 w381]
      tunnel: [_ TRUE _ TRUE] -> w366
      tunnel: [w369 w373 w377 _] -> w365
      tunnel: [w368 w372 w378 w381] -> w364
      event "Start": Value Change {
        n137 = event-data() -> ()  [unwired: 1 in, 1 out]
        n138 = call "Enqueue Message.vi"("Message"="Start Acquisition" ("Message 2"), "Queue in"=w371) -> ("error out"=w369:errorcluster, "Queue out"=w368:refnum<queue>)  [unwired: 8 in]
      }
      event "Exit": Value Change {
        n139 = event-data() -> ()  [unwired: 1 in, 1 out]
        n140 = call "Enqueue Message.vi"("Message"="Exit", "Queue in"=w375) -> ("error out"=w373:errorcluster, "Queue out"=w372:refnum<queue>)  [unwired: 8 in]
      }
      event "Stop": Value Change {
        n141 = event-data() -> ()  [unwired: 1 in, 1 out]
        n142 = call "Enqueue Message.vi"("Message"="Stop Acquisition", "Queue in"=w379) -> ("error out"=w377:errorcluster, "Queue out"=w378:refnum<queue>)  [unwired: 8 in]
      }
      event User Event {
        n143 = event-data() -> ()  [unwired: 1 in, 1 out]
        n144 = local write "Display"("\"Exit\" button pressed" ("Message")) -> ()
      }
    }
    n145 = call "Error Handler - Event Handling Loop.vi"("error in (no error)"=w365, "Message Queue"=w364) -> ("dup error in"=w363:errorcluster)  [unwired: 8 in, 1 out]
  }
  n146 = Unregister For Events(event registration refnum=w4, error in=w3) -> (error out=w2:errorcluster)
  n147 = Merge Errors(w2, w9, w1) -> (→"error out":errorcluster)
